vi "Test_Load.vi"() -> ()   [LabVIEW 2019]
uses:
  <vilib>/Palette API/Palette Menu/Public Type Define/View Format.ctl
  <vilib>/Palette API/Palette Menu/Public Type Define/Help Info.ctl
  <vilib>/Palette API/Palette Menu/Public Type Define/Synchronize Info.ctl
  <vilib>/Palette API/Palette Menu/Public Type Define/Palette type.ctl
  <vilib>/Palette API/Palette Menu/Palette Menu.lvlib
panel:
  out "palette data":T4={"display name"="", "view format"=2, "palette width"=0, "items"=[], "256 color icon"=bytes[0], "B&W color icon"=bytes[0], "help information"={"help tag"="", "help file path "=path ""}, "palette description"="", "synchronize information"={"synchronize with directory"=FALSE, "synchronize directory path"=path ""}} {"view format" items=["Icons", "Text", "Icons and Text"]}
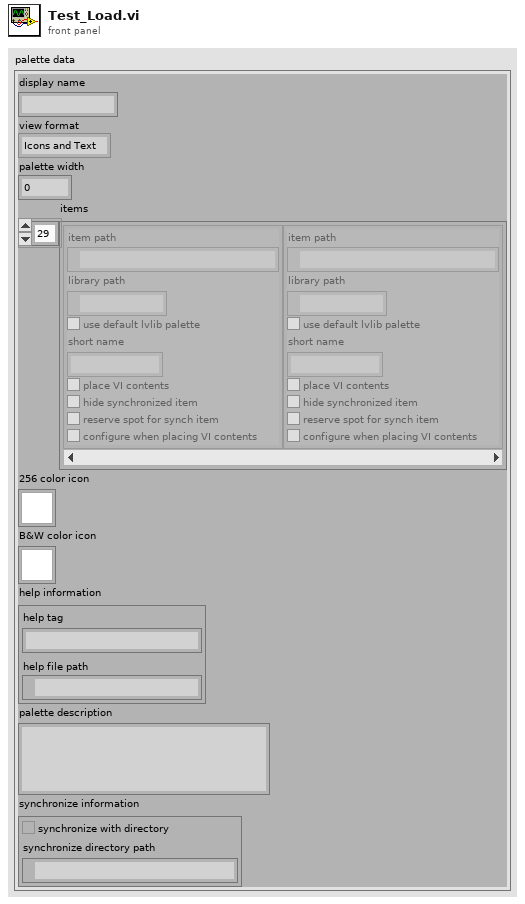
[diagram p1: front panel]
types:
  T1 = typedef "Palette Menu.lvlib/View Format.ctl" = u16
  T2 = typedef "Palette Menu.lvlib/Help Info.ctl" = cluster{"help tag":string, "help file path ":path}
  T3 = typedef "Palette Menu.lvlib/Synchronize Info.ctl" = cluster{"synchronize with directory":bool, "synchronize directory path":path}
  T4 = cluster{"display name":string, "view format":T1, "palette width":i16, "items":cluster{"item path":path, "library path":path, "use default lvlib palette":bool, "short name":string, "place VI contents":bool, "hide synchronized item":bool, "reserve spot for synch item":bool, "configure when placing VI contents":bool}[], "256 color icon":picture, "B&W color icon":picture, "help information":T2, "palette description":string, "synchronize information":T3}
  T5 = typedef "Palette Menu.lvlib/Palette type.ctl" = i32
  T6 = typedef "Palette Menu.lvlib/Palette Data.ctl" = cluster{"display name":string, "view format":T1, "palette width":i16, "items":T7, "256 color icon":picture, "B&W color icon":picture, "help information":T2, "palette description":string, "synchronize information":T3}
  T7 = typedef "Palette Menu.lvlib/Items.ctl" = T8[]
  T8 = typedef "Palette Menu.lvlib/Item.ctl" = cluster{"item path":path, "library path":path, "use default lvlib palette":bool, "short name":string, "place VI contents":bool, "hide synchronized item":bool, "reserve spot for synch item":bool, "configure when placing VI contents":bool}
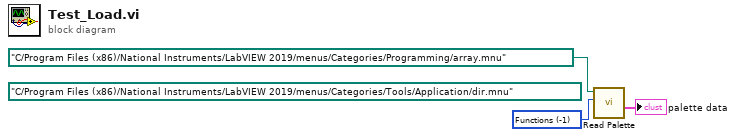
[diagram p0: block diagram]
diagram:
  w3 = T5 -1 items=["Functions"=-1, "Controls"=-2] ("palette type")
  (unwired) path "C:/Program Files (x86)/National Instruments/LabVIEW 2019/menus/Categories/Tools/Application/dir.mnu" ("palette path")
  n1 = call <vilib>:"Read Palette.vi"("palette type"=w3, "palette path"=path "C:/Program Files (x86)/National Instruments/LabVIEW 2019/menus/Categories/Programming/array.mnu") -> ("palette data"=→"palette data":T6)  [unwired: 7 in, 2 out]
